vi "ConvertMeasureToVoltage.vi"(1 "Input Measure":u16) -> (0 "Voltage":dbl)   [LabVIEW 2021]
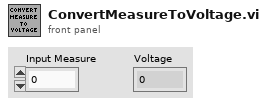
[diagram p1: front panel]
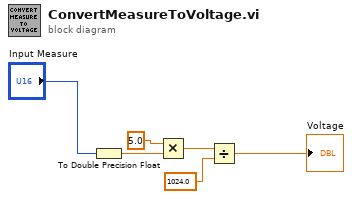
[diagram p0: block diagram]
diagram:
  n1 = To Double Precision Float(number="Input Measure") -> (double precision float=w5:dbl)
  n2 = Multiply(x=5.0, y=w5) -> (x*y=w2:dbl)
  n3 = Divide(x=w2, y=1024.0) -> (x/y=→"Voltage":dbl)
